vi "SPC_stream_reset.vi"(6 "Stream Handle":i16, 8 "Error In":errorcluster, 11 "DLL Path":path) -> (0 "Error Out":errorcluster, 3 "DLL Path":path, 4 "Stream Handle":i16)   [LabVIEW 2017]
doc: "The procedure resets buffered stream ‘stream_hndl’ to the state before extracting the photons without affecting stream’s internal data buffers. After this user can define new stream’s start/stop condition and extract photons once more from the beginning of the stream using new conditions. But, attention, this is possible only when stream’s data buffers are not freed after extracting photons.\n\nAn option FREE_BUF_STREAM ( bit 13 in ‘stream_type’ parameter while initializing the stream using SPC_init_buf_stream function) defines a way in which stream’s buffers are freed. If it is set, the buffer is freed, when, during SPC_get_photons_from_stream call, all photons from the current buffer are extracted. \n\nAfter this it will be not possible to use the buffer again, for example to get data from it using SPC_get_buffer_from_stream function. Therefore SPC_reset_stream can be used when FREE_BUF_STREAM is not used – buffers are not freed and extracting photons can be repeated.\n\ninfo@becker-hickl.com"
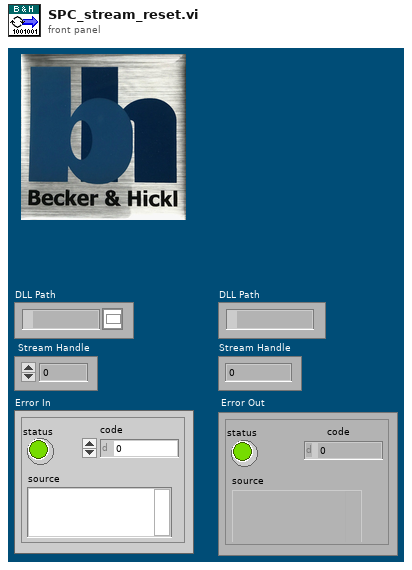
[diagram p1: front panel]
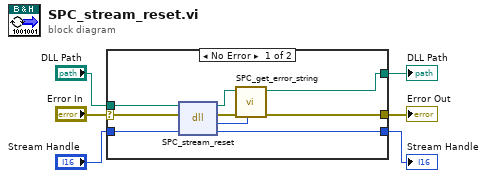
[diagram p0: block diagram]
diagram:
  n1 = case shown="No Error" "Error In" {
    selector: "Error In" -> [w12 w18]
    tunnel: "DLL Path" -> [w15 w17]
    tunnel: [w10 w17] -> w5
    tunnel: [w13 w18] -> w4
    tunnel: "Stream Handle" -> [w8 w16]
    tunnel: [w7 w16] -> w1
    frame No Error {
      n2 = dll-call lib="D:/spcm/lib/lab_view/lv10.0/spcm32.dll" fn="SPC_stream_reset"(path in=w15, error in=w12, "stream_hndl"=w8) -> (path out=w11:path, error out=w14:errorcluster, "return type"=w9:i16, "stream_hndl"=w7:i16)  [unwired: 1 in]
      n3 = call "SPC_get_error_string.vi"("ErrorID"=w9, "Error In"=w14, "DLL Path"=w11) -> ("Error Out"=w13:errorcluster, "DLL Path"=w10:path)  [unwired: 6 in, 1 out]
    }
    frame Error {
    }
  }
  "DLL Path" <- w5
  "Error Out" <- w4
  "Stream Handle" <- w1
